vi "4.2 Surface Area and Volume of a Sphere-Prob3.vi"() -> ()   [LabVIEW 2025]
panel:
  out "MIN Resistance":dbl
  out "MAX Resistance":dbl
  in  "Tolerance in %":dbl
  in  "Resistance Value":dbl
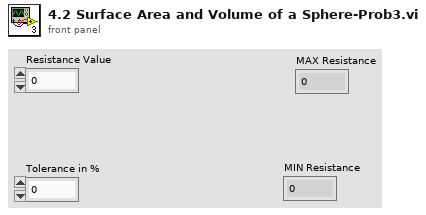
[diagram p1: front panel]
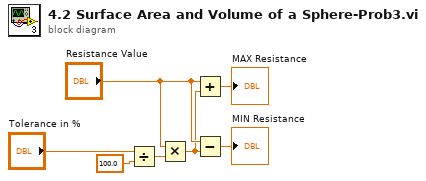
[diagram p0: block diagram]
diagram:
  n1 = Divide(x="Tolerance in %", y=100.0) -> (x/y=w5:dbl)
  n2 = Multiply(x="Resistance Value", y=w5) -> (x*y=w2:dbl)
  n3 = Add(x="Resistance Value", y=w2) -> (x+y=→"MAX Resistance":dbl)
  n4 = Subtract(x="Resistance Value", y=w2) -> (x-y=→"MIN Resistance":dbl)
